vi "Fdx Stop (Rx).vi"(8 "error in":errorcluster, 10 "Force Stop?":bool=TRUE, 11 "InstrumentHandle_port in":u32) -> (0 "error out":errorcluster, 3 "InstrumentHandle_port out":u32)   [LabVIEW 2020, in "AIM664LV.lvlib"]
doc: "This function is used to stop the receive operation of the board."
uses:
  AIM664LV.lvlib
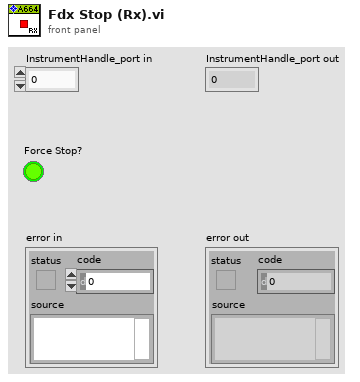
[diagram p1: front panel]
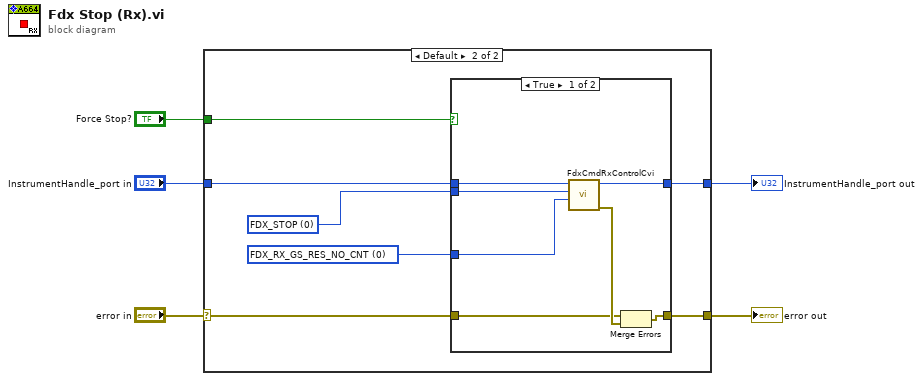
[diagram p0: block diagram]
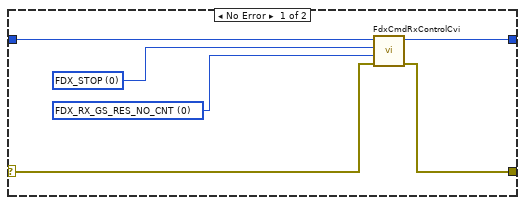
[diagram p2: hidden frame]
diagram:
  n1 = case shown="Default" "error in" {
    selector: "error in" -> [w10 w17]
    tunnel: [w11 w18] -> w1
    tunnel: "Force Stop?" -> [_ w16]
    tunnel: [w9 w15] -> w3
    tunnel: "InstrumentHandle_port in" -> [w8 w14]
    frame No Error {
      w7 = u32 0 items=["FDX_STOP", "FDX_START"] ("StartMode")
      w6 = u32 0 items=["FDX_RX_GS_RES_NO_CNT", "FDX_RX_GS_RES_ALL_CNT", "FDX_RX_GS_RES_ERR_CNT "] ("GlobalStatisticReset")
      n2 = call "FdxCmdRxControlCvi.vi"("error in"=w10, "GlobalStatisticReset"=w6, "StartMode"=w7, "InstrumentHandle_port in"=w8) -> ("error out"=w11:errorcluster, "InstrumentHandle_port out"=w9:u32)  [unwired: 6 in]
    }
    frame Default {
      w13 = u32 0 items=["FDX_STOP", "FDX_START"] ("StartMode")
      w12 = u32 0 items=["FDX_RX_GS_RES_NO_CNT", "FDX_RX_GS_RES_ALL_CNT", "FDX_RX_GS_RES_ERR_CNT "] ("GlobalStatisticReset")
      n3 = case shown="True" w16 {
        tunnel: [w25 w26] -> w15
        tunnel: [w20 w27] -> w18
        tunnel: w17 -> [w19 w27]
        tunnel: w14 -> [w23 w26]
        tunnel: w13 -> [w22 _]
        tunnel: w12 -> [w21 _]
        frame True {
          n4 = call "FdxCmdRxControlCvi.vi"("GlobalStatisticReset"=w21, "StartMode"=w22, "InstrumentHandle_port in"=w23) -> ("error out"=w24:errorcluster, "InstrumentHandle_port out"=w25:u32)  [unwired: 7 in]
          n5 = Merge Errors(w19, w24) -> (w20:errorcluster)
        }
        frame False {
        }
      }
    }
  }
  "error out" <- w1
  "InstrumentHandle_port out" <- w3
